vi "Subpanel Write Local Error.vi"(8 "error in (no error)":errorcluster, 11 "CIF_UI in":refnum<class "CIF_UI.lvclass">) -> (0 "error out":errorcluster)   [LabVIEW 2021, in "CIF_UI.lvclass"]
uses:
  CIF_UI.lvclass
  CIF_UI.lvclass/CIF_UI.ctl
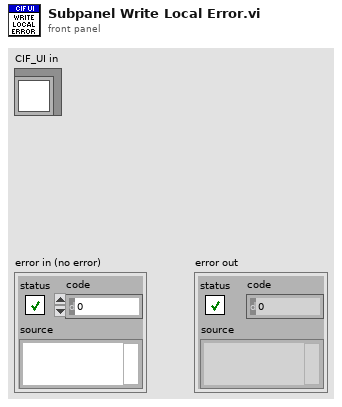
[diagram p1: front panel]
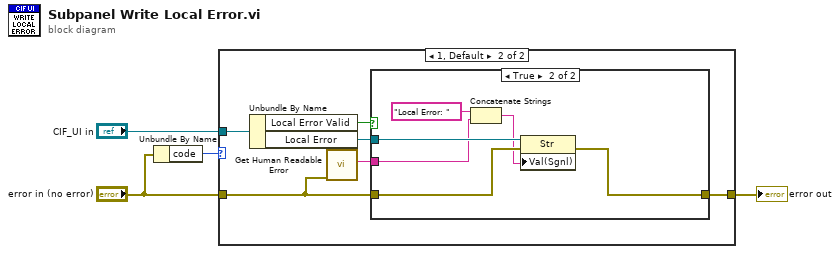
[diagram p0: block diagram]
diagram:
  n1 = Unbundle By Name("error in (no error)") -> ("code"=w1:i32)
  n2 = case shown="1, Default" w1 {
    tunnel: "CIF_UI in" -> [_ w11]
    tunnel: [w5 w8] -> w3
    tunnel: "error in (no error)" -> [w5 w6]
    frame 0 {
    }
    frame 1, Default {
      n3 = Unbundle By Name(w11) -> ("Local Error Valid"=w10:bool, "Local Error"=w9:refnum<vi>)
      n4 = call "Get Human Readable Error.vi"("error in (no error)"=w6) -> ("Error Message"=w7:string)  [unwired: 10 in]
      n5 = case shown="True" w10 {
        tunnel: w9 -> [_ w18]
        tunnel: w7 -> [_ w14]
        tunnel: w6 -> [w12 w17]
        tunnel: [w12 w16] -> w8
        frame False {
        }
        frame True {
          n6 = Concatenate Strings("Local Error: " ("string"), w14) -> (w13:string)
          n7 = property class="Str"(reference=w18, error in=w17, "Val(Sgnl)"=w13) -> (error out=w16:errorcluster)  [unwired: 1 out]
        }
      }
    }
  }
  "error out" <- w3
